vi "Get LL values from String.vi"(11 "input string":string) -> (3 "/limelight/":dbl[](array[numeric]))   [LabVIEW 2020]
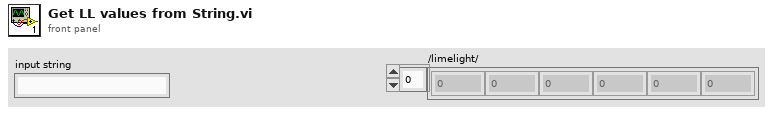
[diagram p1: front panel]
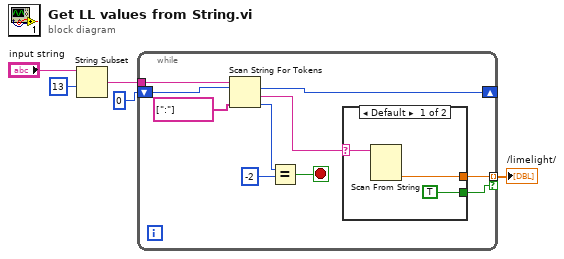
[diagram p0: block diagram]
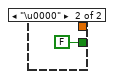
[diagram p2: hidden frame]
diagram:
  n1 = String Subset(string="input string", offset (0)=13) -> (substring=w4:string)  [unwired: 1 in]
  n2 = while {
    tunnel: w4 -> [w12]
    shift-right: [w11] -> _
    shift-left: 0 ("offset past token") -> [w10]
    tunnel: [w7] -> w1 mode=indexing if=w6
    stop <- w15 stop-if-true
    n3 = Scan String For Tokens(6:string[] [":"] ("operators (none)"), 8:w10, 9:w12) -> (0:w14:i32, 1:w8:string, 2:w11:i32)  [unwired: 3 in, 1 out]
    n4 = Equal?(x=w14, y=-2) -> (x = y?=w15:bool)
    n5 = case shown="Default" w8 {
      selector: w8 -> [w17 _]
      tunnel: [w16 _] -> w7
      tunnel: [TRUE FALSE] -> w6
      frame Default {
        n6 = Scan From String(input string=w17) -> (output 1=w16:dbl)  [unwired: 4 in, 3 out]
      }
      frame "\u0000" {
      }
    }
  }
  "/limelight/" <- w1
